vi "1.6.5-mm2in.vi"(1 "mm":i16) -> (0 "in":i16)   [LabVIEW 2010]
doc: "Converts milimeters to Inches"
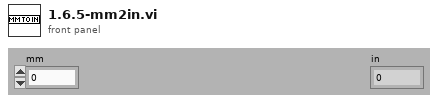
[diagram p1: front panel]
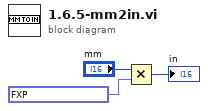
[diagram p0: block diagram]
diagram:
  n1 = Multiply(x="mm", y=fxp<+,16,1> 0.03936767578125) -> (x*y=→"in":i16)
